vi "图形控件之波形图表的使用.vi"() -> ()   [LabVIEW 2018]
panel:
  in  "停止":bool
  out "波形图表":cluster{dbl, dbl}(graph)
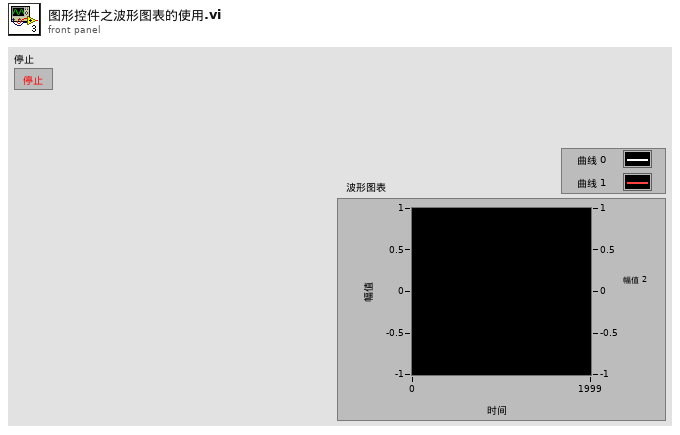
[diagram p1: front panel]
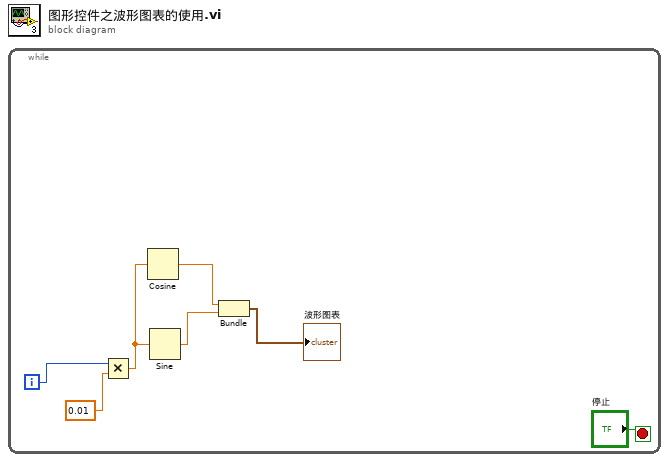
[diagram p0: block diagram]
diagram:
  n1 = while {
    i -> [w5]
    stop <- "停止" stop-if-true
    n2 = Multiply(x=w5, y=0.01) -> (x*y=w4:dbl)
    n3 = Cosine(x=w4) -> (cos(x)=w2:dbl)
    n4 = Sine(x=w4) -> (sin(x)=w3:dbl)
    n5 = Bundle(w2, w3) -> (→"波形图表":cluster{dbl, dbl})  [unwired: 1 in]
  }
